vi "登录.vi"(8 "error in (no error)":errorcluster caption="错误输入（无错误）") -> (0 "error in (no error) 2":errorcluster caption="错误输入（无错误）", 2 "Ground 2":u16(ring) items=["Administrator", "Engineer", "Operator"], 3 "Element 1":string)   [LabVIEW 2017]
uses:
  Picture/UserLogin.ctl
  Global System.vi
panel:
  in  "Main UPH and Login":enum32{"Login"}(tab)
  in  "Ground":u16(ring) items=["Administrator", "Engineer", "Operator"]
  in  "Login":T1
  in  "Password":string
  in  "User Name":string
  out "system time":string
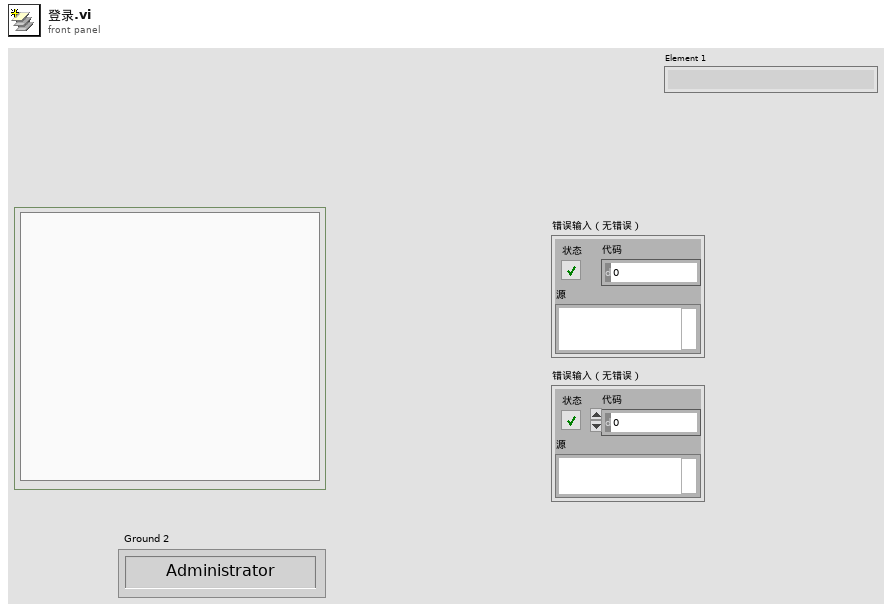
[diagram p1: front panel]
types:
  T1 = typedef "UserLogin.ctl" = bool
  T2 = cluster{"index":i32, "this vi":refnum<vi>, "error out":errorcluster, "用户登录":cluster{"admin":cluster{"用户名":string[], "密码":string[]}, "engineer":cluster{"用户名":string[], "密码":string[]}, "operator":cluster{"用户名":string[], "密码":string[]}}, "用户权限":i32}
  T3 = cluster{"master data":string, "priority":u16, "secondary data":string[]}
  T4 = cluster{"case name":string[], "queue array":refnum<queue>[]}
  T5 = cluster{"admin":cluster{"用户名":string[], "密码":string[]}, "engineer":cluster{"用户名":string[], "密码":string[]}, "operator":cluster{"用户名":string[], "密码":string[]}}
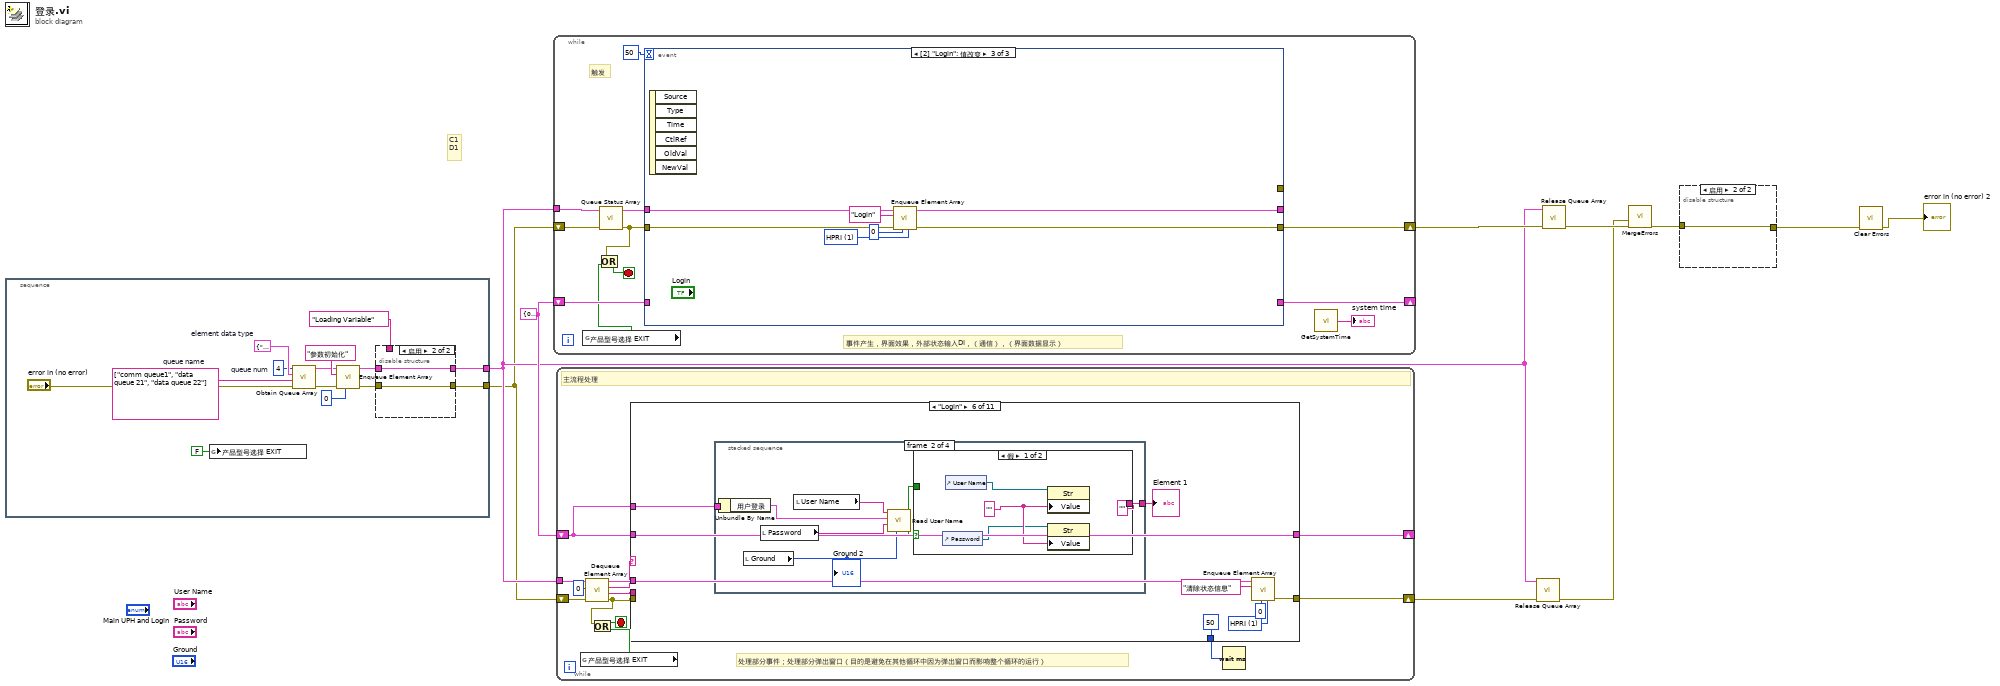
[diagram p0: block diagram]
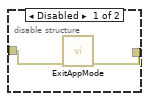
[diagram p2: hidden frame]
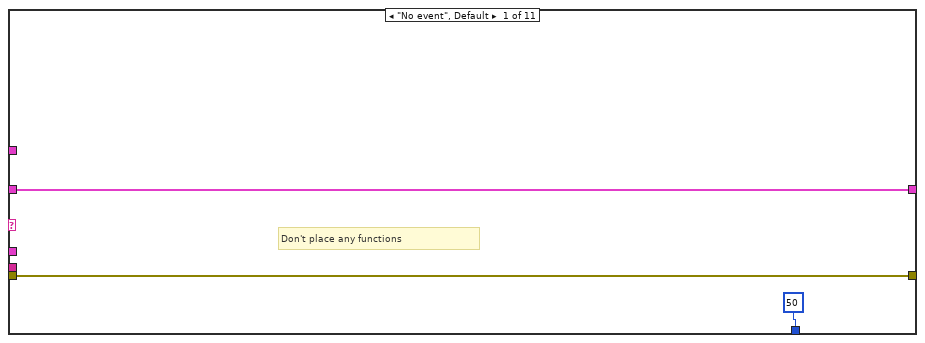
[diagram p3: hidden frame]
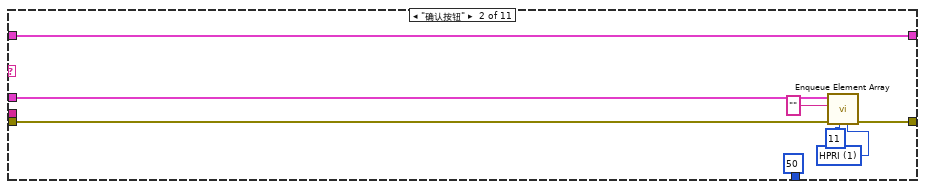
[diagram p4: hidden frame]
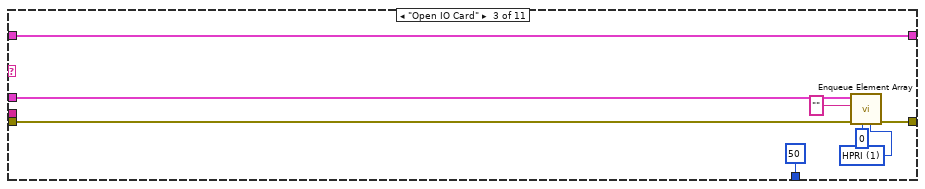
[diagram p5: hidden frame]
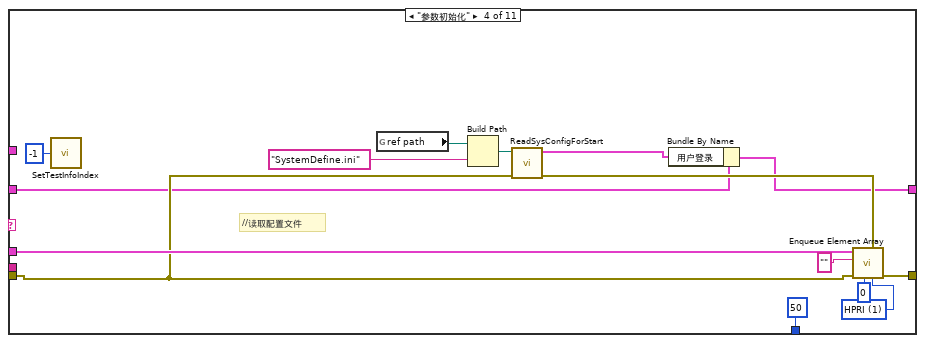
[diagram p6: hidden frame]
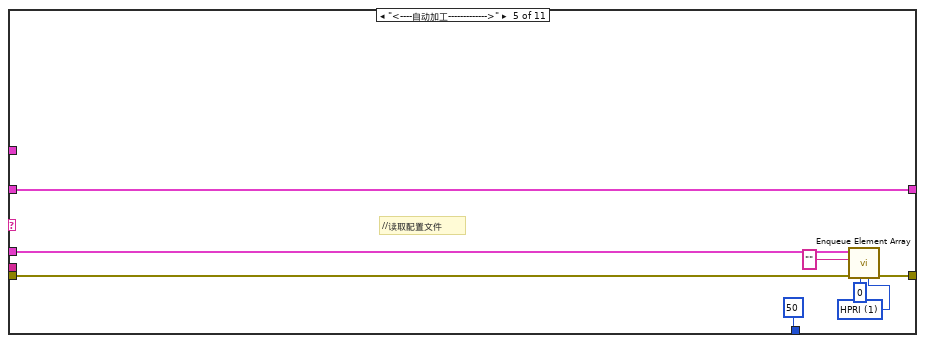
[diagram p7: hidden frame]
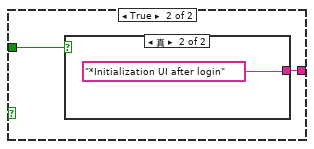
[diagram p9: hidden frame]
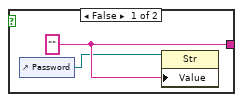
[diagram p10: hidden frame]
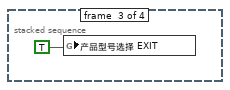
[diagram p11: hidden frame]
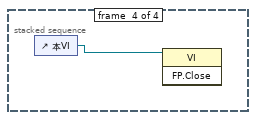
[diagram p12: hidden frame]
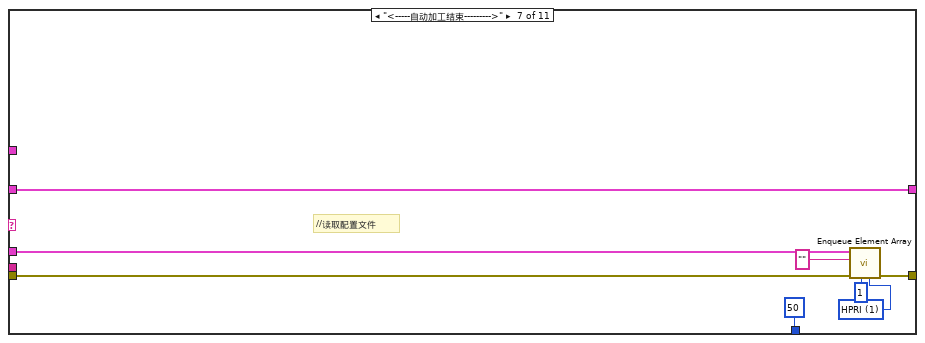
[diagram p13: hidden frame]
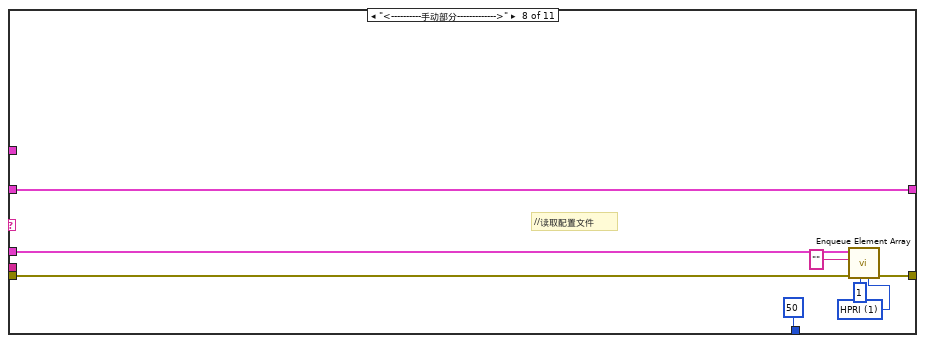
[diagram p14: hidden frame]
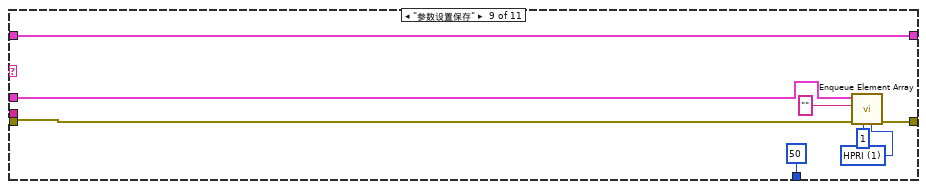
[diagram p15: hidden frame]
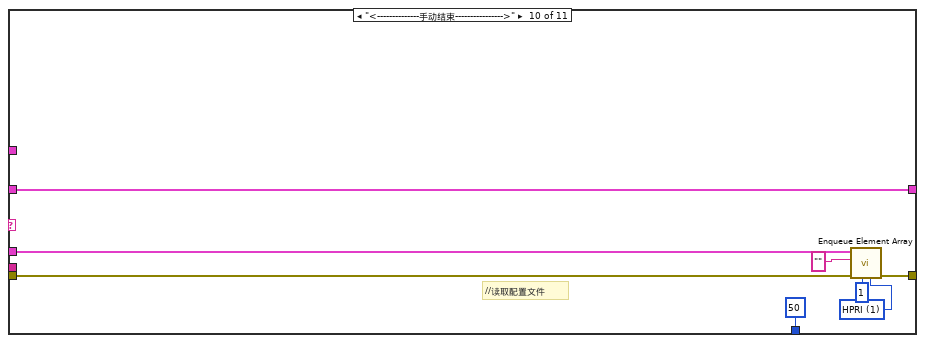
[diagram p16: hidden frame]
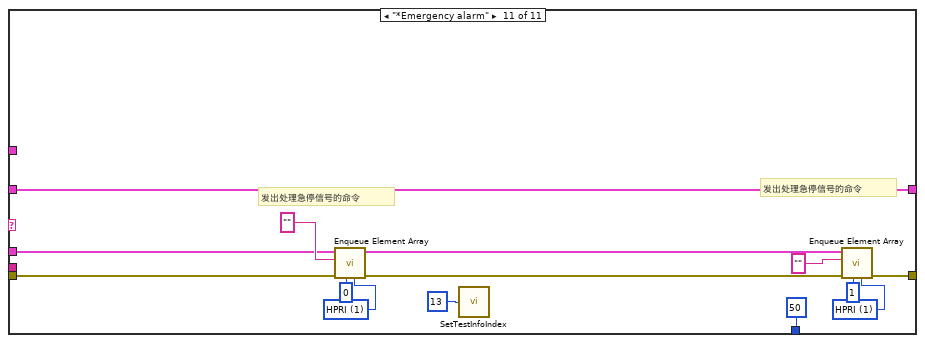
[diagram p17: hidden frame]
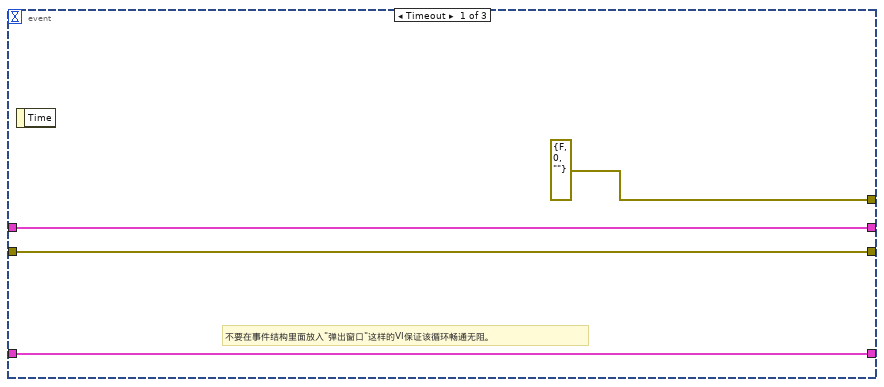
[diagram p18: hidden frame]
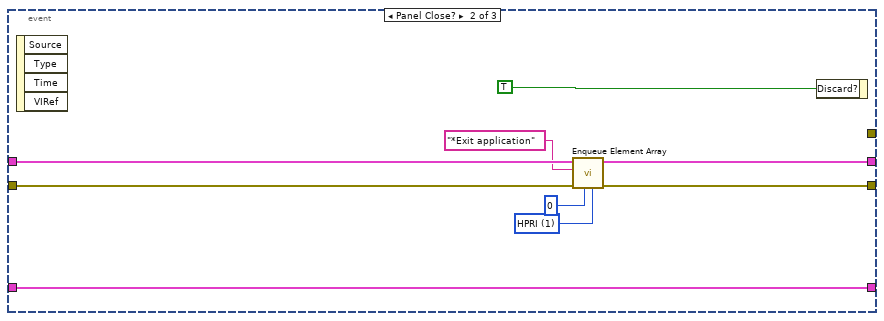
[diagram p19: hidden frame]
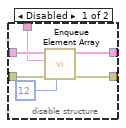
[diagram p20: hidden frame]
diagram:
  w6 = T2 {"index"=0, "this vi"=refnum, "error out"={"status"=FALSE, "code"=0, "source"=""}, "用户登录"={"admin"={"用户名"=[], "密码"=[]}, "engineer"={"用户名"=[], "密码"=[]}, "operator"={"用户名"=[], "密码"=[]}}, "用户权限"=0} ("parameter buffer")
  # "C1\nD1"
  n1 = stacked-sequence {
    tunnel: [w14] -> w2
    tunnel: [w13] -> w3
    frame #0 {
      w22 = string[] ["comm queue1", "data queue 21", "data queue 22"]  # queue name
      w23 = 4  # queue num
      w24 = T3 {"master data"="", "priority"=0, "secondary data"=[]}  # element data type
      n2 = global write "Global System.vi" "产品型号选择 EXIT"(FALSE ("产品型号选择 EXIT")) -> ()
      n3 = call "Obtain Queue Array.vi"("error in (no error)"="error in (no error)", "queue name"=w22, "element data type"=w24, "queue num"=w23) -> ("error out"=w18:errorcluster, "queue out"=w19:T4)  [unwired: 1 in, 1 out]
      n4 = call "Enqueue Element Array.vi"("queue index"=0, "error in"=w18, "master data"="参数初始化", "queue in"=w19) -> ("error out"=w17:errorcluster, "queue out"=w16:T4)  [unwired: 6 in]
      n5 = disable-structure shown="启用" {
        disable-tunnel: w17 -> [w30 w31]
        disable-tunnel: w16 -> [w29 w32]
        disable-tunnel: "Loading Variable" ("master data") -> [w28 _]
        disable-tunnel: [w26 w31] -> w14
        disable-tunnel: [w25 w32] -> w13
        frame Disabled {
          n6 = call "Enqueue Element Array.vi"("queue index"=12, "error in"=w30, "master data"=w28, "queue in"=w29) -> ("error out"=w26:errorcluster, "queue out"=w25:T4)  [unwired: 6 in]
        }
        frame Enabled {
        }
      }
    }
  }
  n7 = while {
    shift-right: [w36] -> w7
    shift-left: w2 -> [w40]
    shift-right: [w38] -> _
    shift-left: w6 -> [w39]
    tunnel: w3 -> [w42]
    stop <- w33 stop-if-true
    # "触发"
    # "事件产生，界面效果，外部状态输入DI，（通信），（界面数据显示）"
    n8 = global read "Global System.vi" "产品型号选择 EXIT"() -> (w34:bool)
    n9 = call "Queue Status Array.vi"("error in (no error)"=w40, "queue in"=w42) -> ("error out"=w35:errorcluster, "queue out"=w37:T4)  [unwired: 4 in]
    n10 = Or(x=w35, y=w34) -> (x .or. y?=w33:bool)
    n11 = event shown="[2] \"Login\": 值改变" {
      selector: _ -> [_ _ _]
      dyn-events: _ -> [_ _ _]
      timeout: 50 -> [_ _ _]
      tunnel: w39 -> [w47 w55 _]
      tunnel: [w47 w55 _] -> w38
      tunnel: [errorcluster {"status"=FALSE, "code"=0, "source"=""} ("error out") _ _] -> _
      tunnel: w37 -> [w45 w54 w60]
      tunnel: w35 -> [w44 w53 w59]
      tunnel: [w44 w52 w57] -> w36
      tunnel: [w45 w51 w58] -> _
      event Timeout {
        # "不要在事件结构里面放入\"弹出窗口\"这样的VI保证该循环畅通无阻。"
        n12 = event-data() -> ()  [unwired: 1 in, 1 out]
      }
      event Panel Close? {
        w49 = u16 1 items=["HPRI"=1, "LPRI"=0] ("priority")
        n13 = event-data() -> ()  [unwired: 1 in, 4 out]
        n14 = call "Enqueue Element Array.vi"("priority"=w49, "queue index"=0, "error in"=w53, "master data"="*Exit application", "queue in"=w54) -> ("error out"=w52:errorcluster, "queue out"=w51:T4)  [unwired: 5 in]
        n15 = event-data("Discard?"=TRUE) -> ()  [unwired: 1 in, 1 out]
      }
      event Value Change {
        w62 = u16 1 items=["HPRI"=1, "LPRI"=0] ("priority")
        n16 = event-data() -> ()  [unwired: 1 in, 6 out]
        n17 = call "Enqueue Element Array.vi"("priority"=w62, "queue index"=0, "error in"=w59, "master data"="Login", "queue in"=w60) -> ("error out"=w57:errorcluster, "queue out"=w58:T4)  [unwired: 5 in]
      }
    }
    n18 = call "GetSystemTime.vi"() -> ("date/time string"=→"system time":string)  [unwired: 7 in]
  }
  n19 = while {
    shift-right: [w76] -> w5
    shift-left: w2 -> [w68]
    shift-right: [w74] -> _
    shift-left: w6 -> [w64]
    tunnel: w3 -> [w70]
    stop <- w65 stop-if-true
    # "处理部分事件；处理部分弹出窗口（目的是避免在其他循环中因为弹出窗口而影响整个循环的运行）"
    # "主流程处理"
    n20 = global read "Global System.vi" "产品型号选择 EXIT"() -> (w66:bool)
    n21 = call "Dequeue Element Array.vi"("queue in"=w70, "queue index"=0, "error in"=w68) -> ("queue out"=w73:T4, "master data"=w72:string, "secondary data"=w71:string[], "error out"=w67:errorcluster)  [unwired: 2 in, 1 out]
    n22 = Or(x=w67, y=w66) -> (x .or. y?=w65:bool)
    n23 = case shown="\"Login\"" w72 {
      tunnel: w73 -> [_ w86 w94 w109 w117 w121 w153 w161 w169 w177 w183]
      tunnel: w67 -> [w78 w82 w90 w100 w113 _ w149 w157 w165 w173 w180]
      tunnel: [w78 w85 w93 w108 w116 w126 w152 w160 w168 w176 w191] -> w76
      tunnel: [50 50 50 50 50 50 50 50 50 50 50] -> w75
      tunnel: w64 -> [w79 w83 w91 w97 w114 w122 w150 w158 w166 w174 w189]
      tunnel: [w79 w83 w91 w96 w114 w122 w150 w158 w166 w174 w189] -> w74
      tunnel: w71 -> [_ _ _ _ _ _ _ _ _ _ _]
      tunnel: w64 -> [_ _ _ _ _ w120 _ _ _ _ _]
      frame "No event", Default {
        # "Don't place any functions"
      }
      frame "确认按钮" {
        w80 = u16 1 items=["HPRI"=1, "LPRI"=0] ("priority")
        n24 = call "Enqueue Element Array.vi"("priority"=w80, "queue index"=11, "error in"=w82, "master data"="" ("Element 1"), "queue in"=w86) -> ("error out"=w85:errorcluster)  [unwired: 5 in, 1 out]
      }
      frame "Open IO Card" {
        w88 = u16 1 items=["HPRI"=1, "LPRI"=0] ("priority")
        n25 = call "Enqueue Element Array.vi"("priority"=w88, "queue index"=0, "error in"=w90, "master data"="" ("Element 1"), "queue in"=w94) -> ("error out"=w93:errorcluster)  [unwired: 5 in, 1 out]
      }
      frame "参数初始化" {
        w105 = u16 1 items=["HPRI"=1, "LPRI"=0] ("priority")
        # "//读取配置文件"
        n26 = call "SetTestInfoIndex.vi"("test info index"=-1) -> ()
        n27 = global read "Global System.vi" "ref path"() -> (w103:path)
        n28 = Build Path ("创建路径")(base path=w103, name or relative path="SystemDefine.ini" ("名称或相对路径")) -> (appended path=w102:path)
        n29 = call "ReadSysConfigForStart.vi"("error in"=w100, "configuration file path"=w102) -> ("error out"=w99:errorcluster, "用户登录"=w98:T5)  [unwired: 8 in]
        n30 = Bundle By Name(cluster=w97, "用户登录"=w98) -> (w96:T2)
        n31 = call "Enqueue Element Array.vi"("priority"=w105, "device error in"=w99, "queue index"=0, "error in"=w100, "master data"="" ("Element 1"), "queue in"=w109) -> ("error out"=w108:errorcluster)  [unwired: 4 in, 1 out]
      }
      frame "<----自动加工------------->" {
        w111 = u16 1 items=["HPRI"=1, "LPRI"=0] ("priority")
        # "//读取配置文件"
        n32 = call "Enqueue Element Array.vi"("priority"=w111, "queue index"=0, "error in"=w113, "master data"="" ("Element 1"), "queue in"=w117) -> ("error out"=w116:errorcluster)  [unwired: 5 in, 1 out]
      }
      frame "Login" {
        w123 = u16 1 items=["HPRI"=1, "LPRI"=0] ("priority")
        n33 = stacked-sequence {
          tunnel: w120 -> [_ w129 _ _]
          tunnel: [_ w128 _ _] -> w119
          frame #0 {
          }
          frame #1 {
            n34 = Unbundle By Name(w129) -> ("用户登录"=w133:T5)
            n35 = local read "Ground"() -> (w130:u16)
            "Ground 2" <- w130
            n36 = local read "Password"() -> (w131:string)
            n37 = local read "User Name"() -> (w132:string)
            n38 = call "Read User Name.vi"("User group"=w130, "Pass word"=w131, "用户登录"=w133, "User name"=w132) -> ("Pass fail"=w134:bool, "User fail"=w135:bool)  [unwired: 6 in]
            n39 = case shown="假" w135 {
              tunnel: w134 -> [_ w141]
              tunnel: ["" ("Element 1") w140] -> w128
              frame False {
                w138 = "" ("User name")
                n40 = control-ref of="Password"() -> (w137:refnum<vi>)
                n41 = control-ref of="User Name"() -> (w136:refnum<vi>)
                n42 = property on="属性节点" class="Str"(reference=w136, "Value"=w138) -> ()  [unwired: 1 in, 2 out]
                n43 = property on="属性节点" class="Str"(reference=w137, "Value"=w138) -> ()  [unwired: 1 in, 2 out]
              }
              frame True {
                n44 = case shown="真" w141 {
                  tunnel: [w143 "*Initialization UI after login" ("Element 1")] -> w140
                  frame False {
                    w143 = "" ("Element 1")
                    n45 = control-ref of="Password"() -> (w142:refnum<vi>)
                    n46 = property on="属性节点" class="Str"(reference=w142, "Value"=w143) -> ()  [unwired: 1 in, 2 out]
                  }
                  frame True {
                  }
                }
              }
            }
          }
          frame #2 {
            n47 = global write "Global System.vi" "产品型号选择 EXIT"(TRUE ("EXIT")) -> ()
          }
          frame #3 {
            n48 = control-ref of="本VI"() -> (w146:refnum<vi>)
            n49 = invoke class="VI" method="FP.Close"(reference=w146) -> ()  [unwired: 2 in, 3 out]
          }
        }
        "Element 1" <- w119
        n50 = call "Enqueue Element Array.vi"("priority"=w123, "queue index"=0, "master data"="清除状态信息" ("Element 1"), "queue in"=w121) -> ("error out"=w126:errorcluster)  [unwired: 6 in, 1 out]
      }
      frame "<-----自动加工结束--------->" {
        w147 = u16 1 items=["HPRI"=1, "LPRI"=0] ("priority")
        # "//读取配置文件"
        n51 = call "Enqueue Element Array.vi"("priority"=w147, "queue index"=1, "error in"=w149, "master data"="" ("Element 1"), "queue in"=w153) -> ("error out"=w152:errorcluster)  [unwired: 5 in, 1 out]
      }
      frame "<----------手动部分------------->" {
        w155 = u16 1 items=["HPRI"=1, "LPRI"=0] ("priority")
        # "//读取配置文件"
        n52 = call "Enqueue Element Array.vi"("priority"=w155, "queue index"=1, "error in"=w157, "master data"="" ("Element 1"), "queue in"=w161) -> ("error out"=w160:errorcluster)  [unwired: 5 in, 1 out]
      }
      frame "参数设置保存" {
        w163 = u16 1 items=["HPRI"=1, "LPRI"=0] ("priority")
        n53 = call "Enqueue Element Array.vi"("priority"=w163, "queue index"=1, "error in"=w165, "master data"="" ("Element 1"), "queue in"=w169) -> ("error out"=w168:errorcluster)  [unwired: 5 in, 1 out]
      }
      frame "<--------------手动结束---------------->" {
        w171 = u16 1 items=["HPRI"=1, "LPRI"=0] ("priority")
        # "//读取配置文件"
        n54 = call "Enqueue Element Array.vi"("priority"=w171, "queue index"=1, "error in"=w173, "master data"="" ("Element 1"), "queue in"=w177) -> ("error out"=w176:errorcluster)  [unwired: 5 in, 1 out]
      }
      frame "*Emergency alarm" {
        w186 = u16 1 items=["HPRI"=1, "LPRI"=0] ("priority")
        w187 = u16 1 items=["HPRI"=1, "LPRI"=0] ("priority")
        # "发出处理急停信号的命令"
        # "发出处理急停信号的命令"
        n55 = call "Enqueue Element Array.vi"("priority"=w186, "queue index"=0, "error in"=w180, "master data"="" ("Element 1"), "queue in"=w183) -> ("error out"=w181:errorcluster, "queue out"=w182:T4)  [unwired: 5 in]
        n56 = call "SetTestInfoIndex.vi"("test info index"=13) -> ()
        n57 = call "Enqueue Element Array.vi"("priority"=w187, "queue index"=1, "error in"=w181, "master data"="" ("Element 1"), "queue in"=w182) -> ("error out"=w191:errorcluster)  [unwired: 5 in, 1 out]
      }
    }
    n58 = Wait (ms)(milliseconds to wait=w75) -> ()  [unwired: 1 out]
  }
  n59 = call "Release Queue Array.vi"("error in"=w5, "queue in"=w3) -> ("error out"=w4:errorcluster)  [unwired: 2 in, 3 out]
  n60 = call "Release Queue Array.vi"("error in"=w7, "queue in"=w3) -> ("error out"=w10:errorcluster)  [unwired: 2 in, 3 out]
  n61 = call "MergeErrors.vi"("error in 3 (no error)"=w4, "error in 4 (no error)"=w10) -> ("error out"=w9:errorcluster)  [unwired: 6 in]
  n62 = disable-structure shown="启用" {
    disable-tunnel: w9 -> [w194 w195]
    disable-tunnel: [w193 w195] -> w8
    frame Disabled {
      n63 = call "ExitAppMode.vi"("error in (no error)"=w194) -> ("error out"=w193:errorcluster)  [unwired: 10 in]
    }
    frame Enabled {
    }
  }
  n64 = call <vilib>:"Clear Errors.vi"("error in (no error)"=w8) -> ("error out"=→"error in (no error) 2":errorcluster)  [unwired: 5 in, 1 out]
